vi "ChromaProtectionStatus.vi"(8 "error in (no error)":errorcluster, 11 "ChromaAcLoad in":refnum<class "ChromaAcLoad.lvclass">) -> (0 "error out":errorcluster, 3 "ChromaAcLoad out":refnum<class "ChromaAcLoad.lvclass">)   [LabVIEW 2018, in "AcPwrPlugins.lvlib" / "ChromaAcLoad.lvclass"]
doc: "This VI retrieves a string status from the Chroma indicating any measurment errors."
uses:
  ChromaAcLoad.lvclass
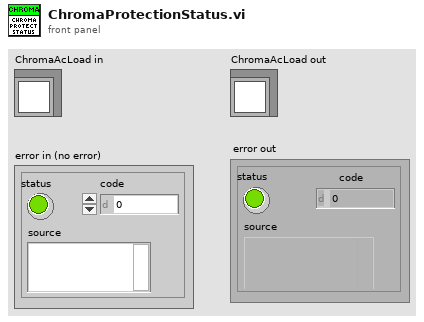
[diagram p1: front panel]
types:
  T1 = typedef "AcPwrPlugins.lvlib/ChromaAcLoad.lvclass/Device(s)Settings.ctl" = cluster{"Configuration Mode":T2, "Phases":cluster{"Handle":string, "Name":string, "Phase Select":i32, "Instrument Options":string, "id query (T)":bool, "reset device (T)":bool, "Load Short Circuited":bool, "Line Synchronization":bool, "Load Current (A/Arms)":dbl, "Load Voltage (V/Vrms)":dbl, "Load Power (W)":dbl, "Load Resistance (Ohms)":dbl, "Load Current Peak Limit (A)":dbl, "Load Current Limit (A/Arms)":dbl, "Load Power Limit (W)":dbl, "Synch Frequency (Hz)":dbl, "Priority":enum16{"CF Only", "PF Only", "Both (CF)", "Both (PF)"}, "Crest Factor":dbl, "Power Factor":dbl, "Slew Rate":cluster{"Rise Slew Rate (A/ms)":i32, "Fall Slew Rate (A/ms)":i32}, "LC/RLC Mode":cluster{"Capacitance (uF)":i32, "Inductance (uH)":i32, "Series Resistance (Ohm)":dbl, "Parallel Resistance (Ohm)":dbl}, "Timing":cluster{"TimingOn":enum16{""}, "Hours":u32, "Minutes":u32, "Seconds":dbl, "CutoffVoltage":dbl}, "Connected":bool}[], "MeasName":string}
  T2 = typedef "ConfigMode.ctl" = enum16{"Constant Voltage (DC)", "Constant Power (DC)", "Constant Power (AC)", "Constant Current (DC)", "Constant Current (AC)", "Constant Resistance (DC)", "Constant Resistance (AC)", "Rectified Mode (DC)", "Inrush (AC)", "RLC CP (AC)", "RLC (AC)"}
  T3 = typedef "AcPwrPlugins.lvlib/ChromaAcLoad.lvclass/Measurements.ctl" = cluster{"Handle":string, "Name":string, "Enabled":bool, "Measurement Value":dbl, "Hold Peak Current Measurement":bool, "btnMeasFetch":bool, "ProtectionStatusString":string, "Measurement Type":T4}[]
  T4 = typedef "AcPwrPlugins.lvlib/ChromaAcLoad.lvclass/MeasurementType.ctl" = enum16{"Voltage (Vrms or V)", "Current (Arms or A)", "Power (W)", "Peak Voltage (V)", "Peak Current (A)", "Peak Power (W)", "Frequency (Hz)", "Resistance (Ohms)", "Voltage Overshoot (V)", "Positive Peak Current (A)", "Voltage Undershoot (V)", "Negative Peak Current (A)", "Apparent Power (VA)", "Reacitive Power (VAR)", "Voltage THD", "Power Factor", "Current's Crest Factor"}
  T5 = cluster{"Handle":string, "Name":string, "Enabled":bool, "Measurement Value":dbl, "Hold Peak Current Measurement":bool, "btnMeasFetch":bool, "ProtectionStatusString":string, "Measurement Type":T4}
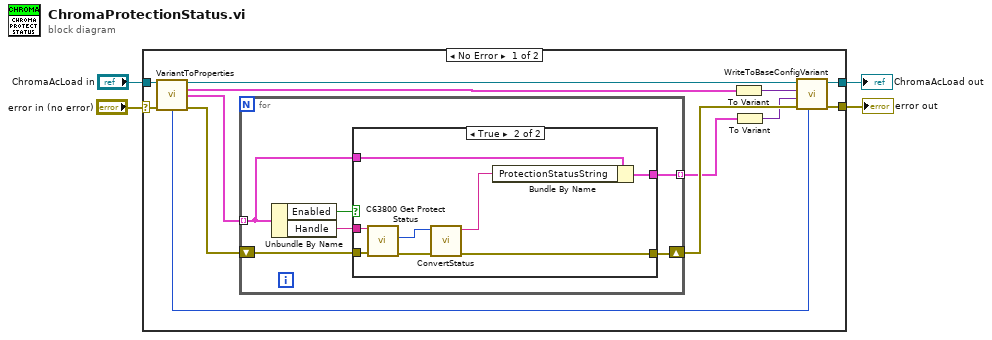
[diagram p0: block diagram]
diagram:
  n1 = case shown="No Error" "error in (no error)" {
    selector: "error in (no error)" -> [w16 w34]
    tunnel: [w12 w35] -> w4
    tunnel: [w10 w34] -> w3
    tunnel: "ChromaAcLoad in" -> [w17 w35]
    frame No Error {
      n2 = call "VariantToProperties.vi"("ChromaAcLoad"=w17, "error in (no error)"=w16) -> ("ChromaAcLoad"=w13:refnum<class "ChromaAcLoad.lvclass">, "Device Properties"=w7:T1, "Meas"=w15:T3, "Measurement Refresh Time (ms)"=w9:u32, "error out"=w14:errorcluster)  [unwired: 7 in, 2 out]
      n3 = for {
        tunnel: w15 -> [w19] mode=indexing
        shift-right: [w22] -> w11
        shift-left: w14 -> [w23]
        tunnel: [w18] -> w6 mode=indexing
        n4 = Unbundle By Name(w19) -> ("Enabled"=w20:bool, "Handle"=w21:string)
        n5 = case shown="True" w20 {
          tunnel: w23 -> [w25 w33]
          tunnel: [w25 w27] -> w22
          tunnel: w21 -> [_ w32]
          tunnel: w19 -> [w24 w31]
          tunnel: [w24 w30] -> w18
          frame False {
          }
          frame True {
            n6 = call <instrlib>:"C63800 Get Protect Status.vi"("error in (no error)"=w33, "Instrument Handle"=w32) -> ("error out"=w29:errorcluster, "Protect Status"=w28:i32)  [unwired: 7 in, 1 out]
            n7 = call "ConvertStatus.vi"("Error In"=w29, "Protect Status"=w28) -> ("Error Out"=w27:errorcluster, "Numeric Indicator"=w26:string)  [unwired: 8 in]
            n8 = Bundle By Name(cluster=w31, "ProtectionStatusString"=w26) -> (w30:T5)
          }
        }
      }
      n9 = To Variant(anything=w7) -> (Variant=w8:variant)
      n10 = To Variant(anything=w6) -> (Variant=w5:variant)
      n11 = call-dynamic "WriteToBaseConfigVariant.vi"("Measurement Refresh Time (ms)"=w9, "error in (no error)"=w11, "Meas"=w5, "Config"=w8, "ChromaAcLoad in"=w13) -> ("error out"=w10:errorcluster, "ChromaAcLoad out"=w12:refnum<class "ChromaAcLoad.lvclass">)  [unwired: 5 in]
    }
    frame Error {
    }
  }
  "ChromaAcLoad out" <- w4
  "error out" <- w3
